vi "Start Async.vi"(8 "error in (no error)":errorcluster, 10 "measurement plugin service in":refnum<class "Measurement Plugin Service.lvclass">, 11 "measurement service v2 in":refnum<class "Measurement Service V2.lvclass">) -> (0 "error out":errorcluster, 3 "measurement service v2 out":refnum<class "Measurement Service V2.lvclass">)   [LabVIEW 2021, in "NI Measurement Plug-In SDK.lvlib" / "Measurement Service V2.lvclass"]
uses:
  Measurement Service V2.lvclass
  C:/Dev/github/ni/measurementlink-labview/Source/Runtime/Measurements/IMeasurement Service/IMeasurement Service.lvclass
  Measurement Plugin Service/Measurement Plugin Service.lvclass
  Measurement Service V2.lvclass/Measurement Service V2.ctl
  IMeasurement Service/IMeasurement Service.lvclass
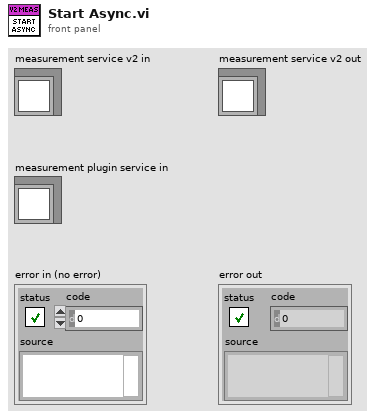
[diagram p1: front panel]
types:
  T1 = typedef "grpc-lvsupport-release.lvlib/grpcId.ctl" = u64
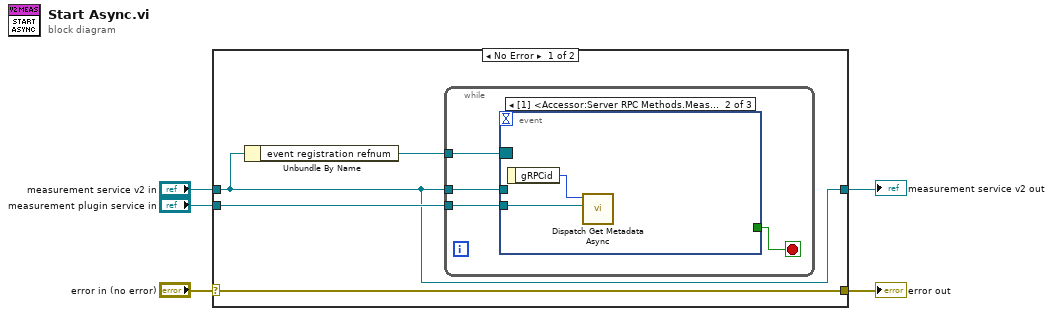
[diagram p0: block diagram]
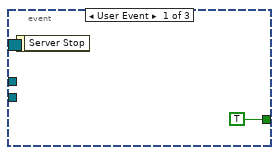
[diagram p2: hidden frame]
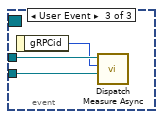
[diagram p3: hidden frame]
diagram:
  n1 = case shown="No Error" "error in (no error)" {
    selector: "error in (no error)" -> [w6 w21]
    tunnel: [w6 w21] -> w4
    tunnel: "measurement plugin service in" -> [w9 _]
    tunnel: "measurement service v2 in" -> [w8 w20]
    tunnel: [w8 w20] -> w3
    frame No Error {
      n2 = Unbundle By Name(w8) -> ("event registration refnum"=w7:refnum<event-registration>)
      n3 = while {
        tunnel: w7 -> [w13]
        tunnel: w9 -> [w12]
        tunnel: w8 -> [w10]
        stop <- w11 stop-if-true
        n4 = event "RPC Methods Event Structure" shown="[1] <Accessor:Server RPC Methods.MeasurementService GetMetadata gRPC UE>: User Event" {
          selector: w13 -> [_ _ _]
          dyn-events: _ -> [_ _ _]
          timeout: _ -> [_ _ _]
          tunnel: [TRUE _ _] -> w11
          tunnel: w12 -> [_ w16 w17]
          tunnel: w10 -> [_ _ w19]
          event User Event {
            n5 = event-data() -> ()  [unwired: 1 in, 1 out]
          }
          event User Event {
            n6 = event-data() -> ("gRPCid"=w15:T1)  [unwired: 1 in]
            n7 = call "Dispatch Get Metadata Async.vi"("measurement plugin service in"=w16, "gRPC ID in"=w15) -> ()  [unwired: 9 in, 1 out]
          }
          event User Event {
            n8 = event-data() -> ("gRPCid"=w18:T1)  [unwired: 1 in]
            n9 = call "Dispatch Measure Async.vi"("measurement plugin service in"=w17, "gRPC ID in"=w18, "measurement service in"=w19) -> ()  [unwired: 8 in, 1 out]
          }
        }
      }
    }
    frame Error {
    }
  }
  "error out" <- w4
  "measurement service v2 out" <- w3
